vi "Launch.vi"(4 "Self":variant, 6 "Parent ID (0)":i32, 7 "VI Path":path, 8 "error in (no error)":errorcluster, 9 "Config Section":string, 10 "Config Path":path, 11 "Name":string) -> (0 "error out":errorcluster, 2 "VI Refnum":refnum<vi>, 3 "Module":T1)   [LabVIEW 2018, in "Core.lvlib" / "Module.lvlib"]
uses:
  Module.lvlib
  Controls/Instance.ctl
  Controls/Module.ctl
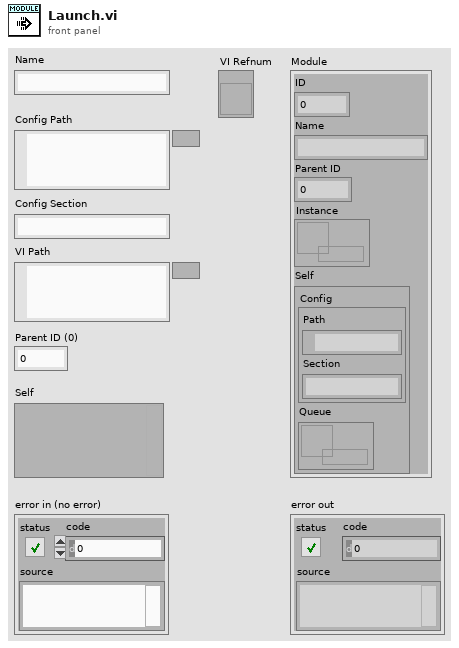
[diagram p1: front panel]
types:
  T1 = typedef "Core.lvlib/Module.lvlib/Module.ctl" = cluster{"ID":i32, "Name":string, "Parent ID":i32, "Instance":refnum<data-value>, "Self":T2}
  T2 = typedef "Core.lvlib/Module.lvlib/Instance.ctl" = cluster{"Config":cluster{"Path":path, "Section":string}, "Queue":refnum<queue>}
  T3 = enum32{"Invalid", "Standard", "Closed", "Hidden", "Minimized", "Maximized"}
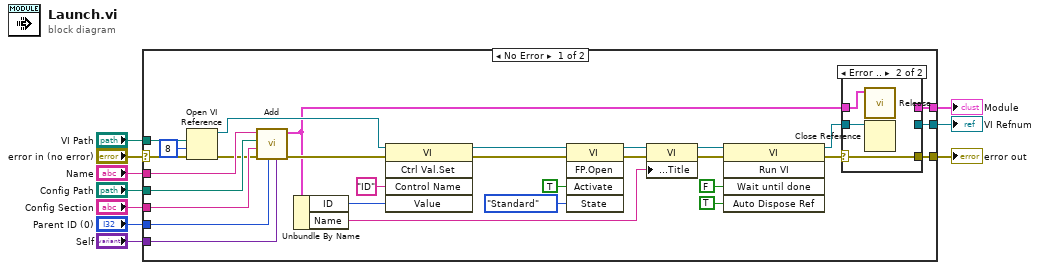
[diagram p0: block diagram]
diagram:
  n1 = case shown="No Error" "error in (no error)" {
    selector: "error in (no error)" -> [w40 w47]
    tunnel: "Parent ID (0)" -> [w18 _]
    tunnel: "Name" -> [w39 _]
    tunnel: "Config Path" -> [w38 _]
    tunnel: "Config Section" -> [w37 _]
    tunnel: [w11 _] -> w5
    tunnel: "VI Path" -> [w34 _]
    tunnel: [w16 w47] -> w3
    tunnel: [w13 _] -> w2
    tunnel: "Self" -> [w17 _]
    frame No Error {
      n2 = Open VI Reference(vi path=w34, options=8, error in (no error)=w40) -> (vi reference=w31:refnum<vi>, error out=w35:errorcluster)  [unwired: 3 in]
      n3 = call "Add.vi"("Self"=w17, "Parent ID (0)"=w18, "error in (no error)"=w35, "Config Section"=w37, "Config Path"=w38, "Name"=w39) -> ("error out"=w36:errorcluster, "Module"=w12:T1)  [unwired: 4 in]
      n4 = Unbundle By Name(w12) -> ("ID"=w29:i32, "Name"=w19:string)
      n5 = invoke class="VI" method="Ctrl Val.Set"(reference=w31, error in=w36, "Control Name"="ID", "Value"=w29) -> (reference out=w27:refnum<vi>, error out=w32:errorcluster)  [unwired: 1 in, 3 out]
      n6 = invoke class="VI" method="FP.Open"(reference=w27, error in=w32, "Activate"=TRUE ("Activate?"), "State"=T3."Standard") -> (reference out=w21:refnum<vi>, error out=w28:errorcluster)  [unwired: 1 in, 3 out]
      n7 = property class="VI"(reference=w21, error in=w28, "Front Panel.Title"=w19) -> (reference out=w20:refnum<vi>, error out=w22:errorcluster)
      n8 = invoke class="VI" method="Run VI"(reference=w20, error in=w22, "Wait until done"=FALSE ("Wait Until Done"), "Auto Dispose Ref"=TRUE ("Auto Dispose Reference")) -> (reference out=w14:refnum<vi>, error out=w15:errorcluster)  [unwired: 1 in, 3 out]
      n9 = case shown="Error .." w15 {
        selector: w15 -> [w43 w46]
        tunnel: [w43 w46] -> w16
        tunnel: w14 -> [w42 w44]
        tunnel: [w42 _] -> w13
        tunnel: w12 -> [w41 w45]
        tunnel: [w41 _] -> w11
        frame No Error {
        }
        frame Error {
          n10 = call "Release.vi"("Module"=w45) -> ()  [unwired: 9 in, 2 out]
          n11 = Close Reference(reference=w44) -> ()  [unwired: 1 in, 1 out]
        }
      }
    }
    frame Error {
    }
  }
  "error out" <- w3
  "Module" <- w5
  "VI Refnum" <- w2
